vi "test.vi"() -> ()   [LabVIEW 2016, in "SeqProcessor.lvlib"]
uses:
  SeqProcessor.lvlib
panel:
  out "value":T1(array[cluster])
  out "JSON string":string
  in  "Sequence":T1(array[cluster])
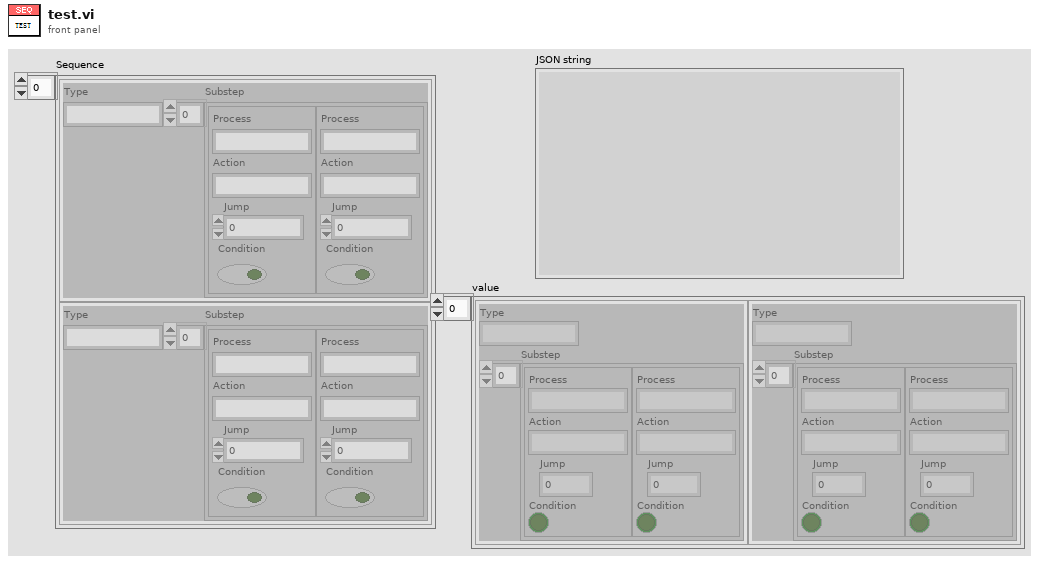
[diagram p1: front panel]
types:
  T1 = cluster{"Type":string, "Substep":cluster{"Process":string, "Action":string, "Jump":i32, "Condition":bool}[]}[]
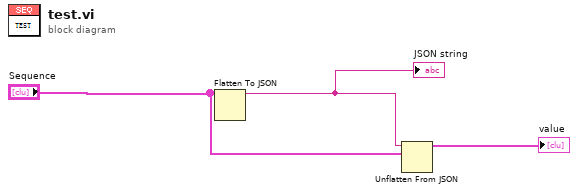
[diagram p0: block diagram]
diagram:
  n1 = Flatten To JSON(anything="Sequence") -> (JSON string=w3:string)  [unwired: 2 in, 1 out]
  "JSON string" <- w3
  n2 = Unflatten From JSON(JSON string=w3, type and defaults="Sequence") -> (value=→"value":T1)  [unwired: 5 in, 1 out]
